vi "RichToFlatRequest.vi"(5 "OutputClusterType":T1, 11 "InputCluster":T2) -> (3 "OutputCluster":T1)   [LabVIEW 2019, in "Generated_server.lvlib"]
uses:
  Generated_server.lvlib
  Request.ctl
  Request_request_oneof/Request_request_oneof.lvclass
  Request_Flat.ctl
  Request_request_oneof/Request_request_oneof.lvclass/Request_request_oneof.ctl
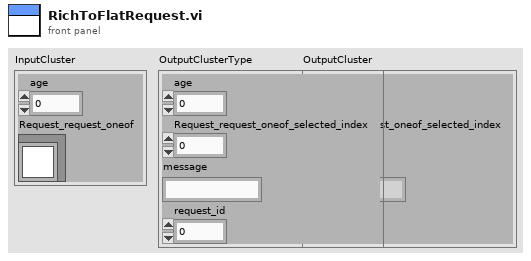
[diagram p1: front panel]
types:
  T1 = typedef "Generated_server.lvlib/Request_Flat.ctl" = cluster{"age":i32, "Request_request_oneof_selected_index":i32, "message":string, "request_id":i32}
  T2 = typedef "Generated_server.lvlib/Request.ctl" = cluster{"age":i32, "Request_request_oneof":refnum<class "Request_request_oneof.lvclass">}
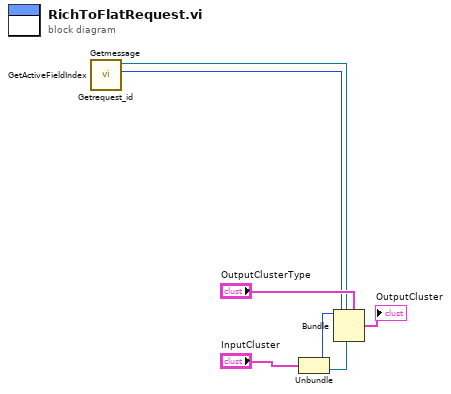
[diagram p0: block diagram]
diagram:
  n1 = Unbundle "Unbundle"("InputCluster") -> ("age"=w5:i32, "Request_request_oneof"=w4:refnum<class "Request_request_oneof.lvclass">)
  n2 = call "Getrequest_id.vi"("OneOfTemplate in"=w4) -> ("Get_Val"=w1:i32)  [unwired: 8 in, 2 out]
  n3 = call "Getmessage.vi"("OneOfTemplate in"=w4) -> ("Get_Val"=w2:string)  [unwired: 8 in, 2 out]
  n4 = call "GetActiveFieldIndex.vi"("OneOfTemplate in"=w4) -> ("Active Field Index"=w3:i32)  [unwired: 8 in, 2 out]
  n5 = Bundle "Bundle"(cluster="OutputClusterType", "age"=w5, "Request_request_oneof_selected_index"=w3, "message"=w2, "request_id"=w1) -> (→"OutputCluster":T1)
